vi "Get Alarm.vi"(8 "error in (no error)":errorcluster, 11 "Motor in":refnum<class "Motor.lvclass">) -> (0 "error out":errorcluster, 2 "Alarm code":i32, 3 "Motor out":refnum<class "Motor.lvclass">)   [LabVIEW 2019, in "Motor.lvclass"]
uses:
  Motor.lvclass
  Motor.lvclass/Motor.ctl
  Motor Serial class/Serial.lvclass
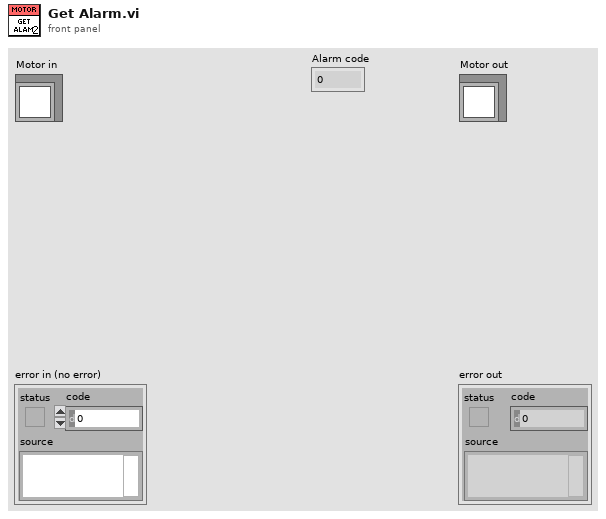
[diagram p1: front panel]
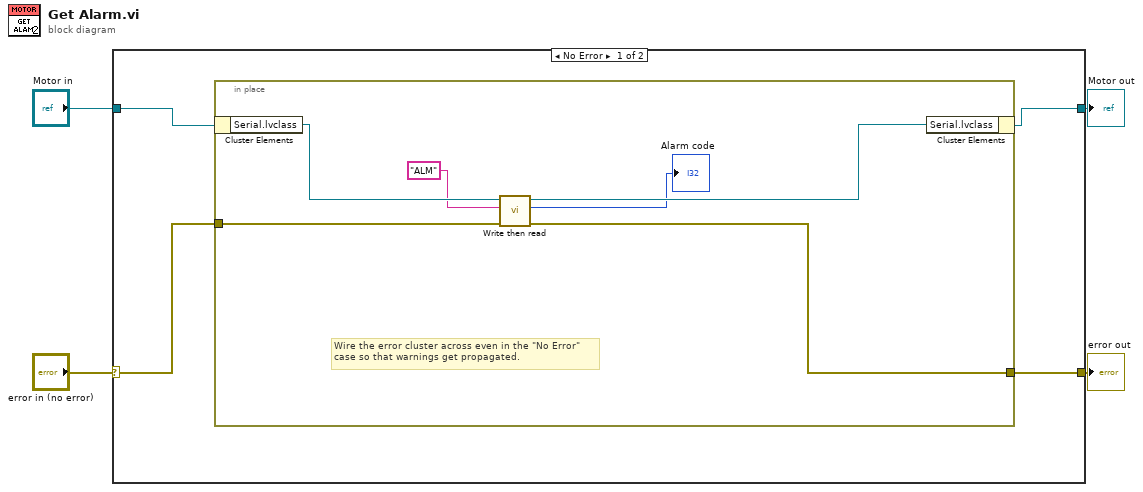
[diagram p0: block diagram]
diagram:
  n1 = case shown="No Error" "error in (no error)" {
    selector: "error in (no error)" -> [w7 w16]
    tunnel: [w6 w16] -> w3
    tunnel: [w8 w15] -> w1
    tunnel: "Motor in" -> [w5 w15]
    frame No Error {
      n2 = in-place {
        in-place-border: w7 -> [w12]
        in-place-border: [w11] -> w6
        # "Wire the error cluster across even in the \"No Error\"\ncase so that warnings get propagated."
        n3 = in-place-cluster #1(w5) -> ("Serial.lvclass"=w14:refnum<class "Serial.lvclass">)
        n4 = call "Write then read.vi"("error in (no error)"=w12, "TX Data"="ALM" ("string"), "Motor_Serial in"=w14) -> ("error out"=w11:errorcluster, "RX Data"=→"Alarm code":i32, "Motor_Serial out"=w13:refnum<class "Serial.lvclass">)  [unwired: 5 in]
        n5 = in-place-cluster #1("Serial.lvclass"=w13) -> (w8:refnum<class "Motor.lvclass">)
      }
    }
    frame Error {
    }
  }
  "error out" <- w3
  "Motor out" <- w1
